vi "DAC_manual_set.vi"() -> ()   [LabVIEW 2013]
uses:
  <vilib>/FPGAPlugInAG/sbRIO-9612/niLvFpga_Close_sbRIO-9612.vi
  <vilib>/rvi/interface/nirviCloseFPGA/nirviCloseFPGA.xnode
  fpga-bitfile-ref.ctl
  FPGA Bitfiles/fpgabatch18_sbRIO9612RIO0_FPGAMAINlock-in_BbNldMosBaM.lvbitx
panel:
  out "moving":bool
  in  "FPGA param":T1={"IP Adress FPGA"="192.168.137.11", "Delay(ms)"=1, "Busses to use"=[TRUE, TRUE, TRUE, TRUE, TRUE, TRUE, TRUE, TRUE], "max"=5.0, "min"=-5.0}
  in  "Read":bool
  in  "Set":bool
  in  "Ramp":bool
  in  "All to":bool
  in  "All to":dbl
  in  "stop":bool
  in  "DAC control":dbl[][](array[numeric])=[[-0.1, -0.2, -0.3, -0.4, -0.5, -0.6, -0.7, -0.8], [0.0, 0.0, 0.0, 0.0, 0.0, 0.0, 0.0, 0.0], [0.0, 0.0, 0.0, 0.0, 0.0, 0.0, 0.0, 0.0], [0.0, 0.0, 0.0, 0.0, 0.0, 0.0, 0.0, 0.0], [0.0, 0.0, 0.0, 0.0, 0.0, 0.0, 0.0, 0.0], [0.0, 0.0, 0.0, 0.0, 0.0, 0.0, 0.0, 0.0], [0.0, 0.0, 0.0, 0.0, 0.0, 0.0, 0.0, 0.0], [-1.1, -1.2, -1.3, -1.4, -1.5, -1.6, -1.7, -1.8]]
  # "All to"
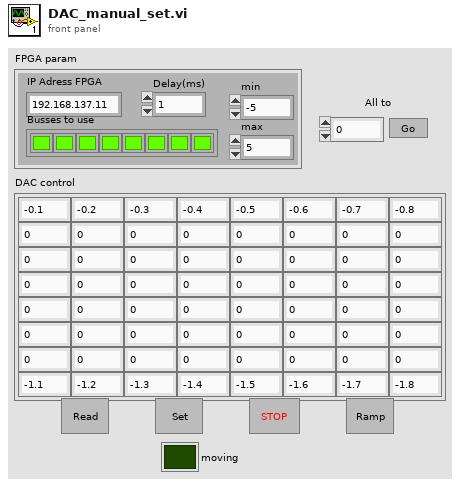
[diagram p1: front panel]
types:
  T1 = cluster{"IP Adress FPGA":string, "Delay(ms)":u8, "Busses to use":bool[], "max":dbl, "min":dbl}
  T2 = enum8{"start movement", "buses to use", "delay", "value", "stop", ""}
  T3 = enum8{"start movement", "buses to use", "delay", "value"}
  T4 = typedef "fpga-bitfile-ref.ctl" = refnum<k20>
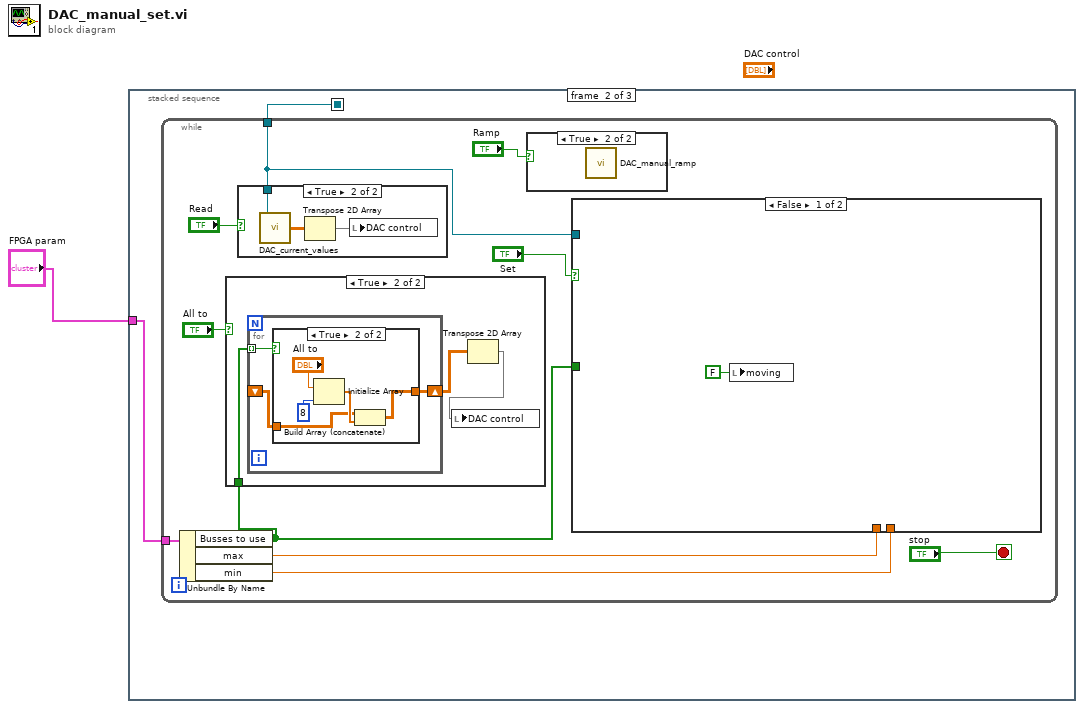
[diagram p0: block diagram]
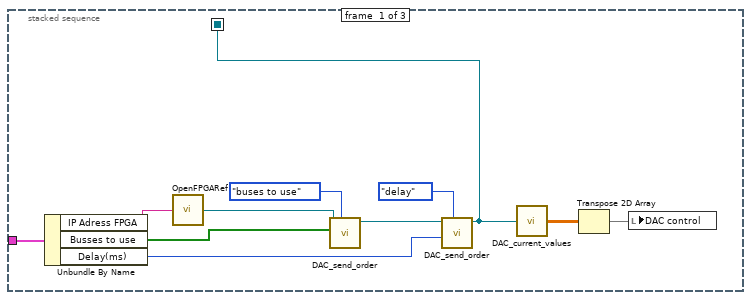
[diagram p2: hidden frame]
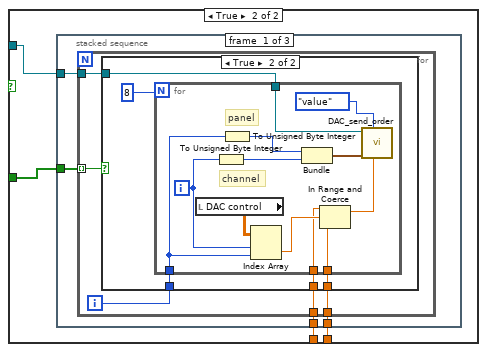
[diagram p4: hidden frame]
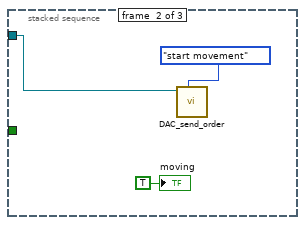
[diagram p6: hidden frame]
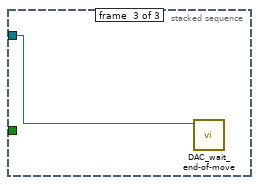
[diagram p7: hidden frame]
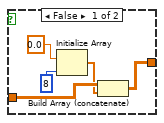
[diagram p9: hidden frame]
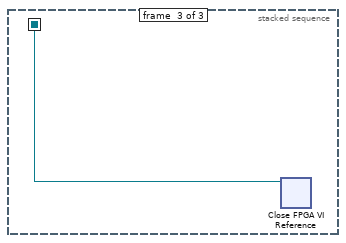
[diagram p11: hidden frame]
diagram:
  n1 = stacked-sequence {
    seq-local: [w8 _ _] -> [_ w14 w79]
    tunnel: "FPGA param" -> [w4 w13 _]
    frame #0 {
      n2 = Unbundle By Name(w4) -> ("IP Adress FPGA"=w5:string, "Busses to use"=w3:bool[], "Delay(ms)"=w2:u8)
      n3 = call "OpenFPGARef.vi"("IP Address"=w5) -> ("FPGA VI Reference Out"=w9:T4)
      n4 = call "DAC_send_order.vi"("order"=T2."buses to use", "buses to use"=w3, "FPGA VI Reference In"=w9) -> ("FPGA VI Reference Out"=w10:T4)  [unwired: 8 in]
      n5 = call "DAC_send_order.vi"("order"=T2."delay", "delay between steps (ms)"=w2, "FPGA VI Reference In"=w10) -> ("FPGA VI Reference Out"=w8:T4)  [unwired: 8 in]
      n6 = call "DAC_current_values.vi"("FPGA Ref"=w8) -> ("DAC values"=w7:sgl[][])
      n7 = Transpose 2D Array(2D array=w7) -> (transposed array=w6:sgl[][])
      n8 = local write "DAC control"(w6) -> ()
    }
    frame #1 {
      n9 = while {
        tunnel: w14 -> [w16]
        tunnel: w13 -> [w20]
        stop <- "stop" stop-if-true
        n10 = Unbundle By Name(w20) -> ("Busses to use"=w19:bool[], "max"=w18:dbl, "min"=w17:dbl)
        n11 = case shown="True" "All to" {
          tunnel: w19 -> [_ w60]
          frame False {
          }
          frame True {
            n12 = for {
              shift-right: [w65] -> w62
              shift-left: _ -> [w64]
              tunnel: w60 -> [w63] mode=indexing
              n13 = case shown="True" w63 {
                tunnel: [w68 w73] -> w65
                tunnel: w64 -> [w69 w71]
                frame False {
                  n14 = Initialize Array(0.0, 8) -> (w67:dbl[])
                  n15 = Build Array (concatenate)(w69, w67) -> (w68:dbl[][])
                }
                frame True {
                  n16 = Initialize Array("All to", 8) -> (w74:dbl[])
                  n17 = Build Array (concatenate)(w71, w74) -> (w73:dbl[][])
                }
              }
            }
            n18 = Transpose 2D Array(2D array=w62) -> (transposed array=w61:dbl[][])
            n19 = local write "DAC control"(w61) -> ()
          }
        }
        n20 = case shown="True" "Read" {
          tunnel: w16 -> [_ w78]
          frame False {
          }
          frame True {
            n21 = call "DAC_current_values.vi"("FPGA Ref"=w78) -> ("DAC values"=w76:sgl[][])
            n22 = Transpose 2D Array(2D array=w76) -> (transposed array=w77:sgl[][])
            n23 = local write "DAC control"(w77) -> ()
          }
        }
        n24 = case shown="True" "Ramp" {
          frame False {
          }
          frame True {
            n25 = call "DAC_manual_ramp.vi"() -> ()  [unwired: 4 in]
          }
        }
        n26 = case shown="False" "Set" {
          tunnel: w16 -> [_ w29]
          tunnel: w19 -> [_ w28]
          tunnel: w18 -> [_ w27]
          tunnel: w17 -> [_ w26]
          frame False {
            n27 = local write "moving"(FALSE ("moving")) -> ()
          }
          frame True {
            n28 = stacked-sequence {
              tunnel: w29 -> [w33 w57 w59]
              tunnel: w28 -> [w32 _ _]
              tunnel: w27 -> [w31 _ _]
              tunnel: w26 -> [w30 _ _]
              frame #0 {
                n29 = for {
                  tunnel: w33 -> [w38]
                  tunnel: w32 -> [w36] mode=indexing
                  tunnel: w31 -> [w35]
                  tunnel: w30 -> [w34]
                  i -> [w37]
                  n30 = case shown="True" w36 {
                    tunnel: w38 -> [_ w43]
                    tunnel: w37 -> [_ w41]
                    tunnel: w35 -> [_ w40]
                    tunnel: w34 -> [_ w39]
                    frame False {
                    }
                    frame True {
                      n31 = for {
                        N: 8 -> [_]
                        tunnel: w43 -> [w50]
                        tunnel: w41 -> [w47]
                        tunnel: w40 -> [w45]
                        tunnel: w39 -> [w44]
                        i -> [w48]
                        # "channel"
                        # "panel"
                        n32 = local read "DAC control"() -> (w49:dbl[][])
                        n33 = To Unsigned Byte Integer(number=w48) -> (unsigned 8bit integer=w53:u8)
                        n34 = To Unsigned Byte Integer(number=w47) -> (unsigned 8bit integer=w54:u8)
                        n35 = Index Array(array=w49, index (row)=w48, index (col)=w47) -> (element=w46:dbl)
                        n36 = Bundle(w54, w53) -> (w52:cluster{u8, u8})  [unwired: 1 in]
                        n37 = In Range and Coerce(upper limit=w45, x=w46, lower limit=w44) -> (coerced(x)=w51:dbl)  [unwired: 1 out]
                        n38 = call "DAC_send_order.vi"("DAC goto value"=w51, "order"=T3."value", "Cluster"=w52, "FPGA VI Reference In"=w50) -> ()  [unwired: 3 in, 5 out]
                      }
                    }
                  }
                }
              }
              frame #1 {
                n39 = call "DAC_send_order.vi"("order"=T3."start movement", "FPGA VI Reference In"=w57) -> ()  [unwired: 5 in, 5 out]
                "moving" <- TRUE ("moving")
              }
              frame #2 {
                n40 = call "DAC_wait_end-of-move.vi"("FPGA VI Reference In"=w59) -> ()  [unwired: 10 in, 1 out]
              }
            }
          }
        }
      }
    }
    frame #2 {
      n41 = xnode "Close FPGA VI Reference"("FPGA VI Reference In"=w79) -> ()  [unwired: 1 in, 1 out]
    }
  }
